vi "Save Recall Instrument Settings.vi"(8 "error in (no error)":errorcluster, 9 "Memory Location (1)":dbl=1.0 min=1.0 max=36.0 format="%#_0f", 10 "Save Recall Settings (0:Save)":i32(ring) items=["Save", "Recall"], 11 "VISA resource name":refnum<visa-resource-name>) -> (0 "error out":errorcluster, 3 "VISA resource name out":refnum<visa-resource-name>)   [LabVIEW 2017, in "BK Precision 913XX.lvlib"]
doc: "Saves or recalls instrument settings to or from a specified memory location.\n\n<b>Note: This vi cannot be used when series, parallel, or tracking mode is enabled. Use Configure Series.vi, Configure Parallel.vi, or Configure Tracking.vi respectively to disable.</b>"
uses:
  <instrlib>/BK Precision 913XX/BK Precision 913XX.lvlib
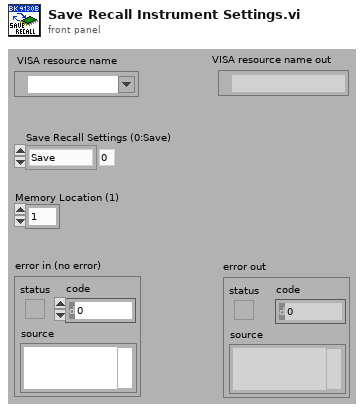
[diagram p1: front panel]
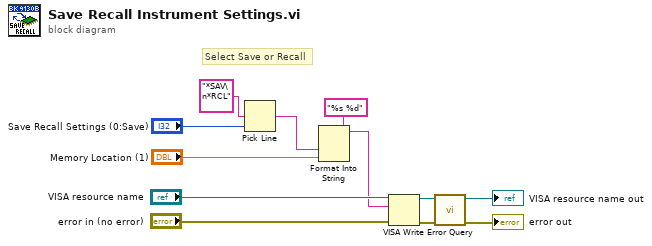
[diagram p0: block diagram]
diagram:
  # "Select Save or Recall"
  n1 = Pick Line(multi-line string="*SAV\n*RCL", line index="Save Recall Settings (0:Save)") -> (output string=w9:string)  [unwired: 1 in]
  n2 = Format Into String(format string="%s %d", w9, "Memory Location (1)") -> (resulting string=w2:string)  [unwired: 2 in, 1 out]
  n3 = VISA Write(VISA resource name="VISA resource name", write buffer=w2, error in (no error)="error in (no error)") -> (VISA resource name out=w5:refnum<visa-resource-name>, error out=w6:errorcluster)  [unwired: 1 out]
  n4 = call <instrlib>:"Error Query.vi"("error in (no error)"=w6, "VISA resource name"=w5) -> ("error out"=→"error out":errorcluster, "VISA resource name out"=→"VISA resource name out":refnum<visa-resource-name>)  [unwired: 6 in, 2 out]
